vi "Command_Turret_AutoTarget.vi"(7 "Startup":bool, 8 "Timeout":dbl, 9 "Kd":dbl, 10 "Ki":dbl, 11 "Kp":dbl) -> (2 "Turret_Speed":dbl, 4 "Reint":bool, 6 "Completed":bool)   [LabVIEW 2019]
uses:
  Auto Utilities/Command_Execution_State.ctl
  Subsystems/Sensing/Sensor_Values.vi
panel:
  in  "Acceptable_Error":dbl
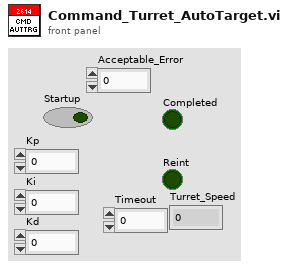
[diagram p1: front panel]
types:
  T1 = typedef "Command_Execution_State.ctl" = enum16{"Initialize", "Execute", "Finish"}
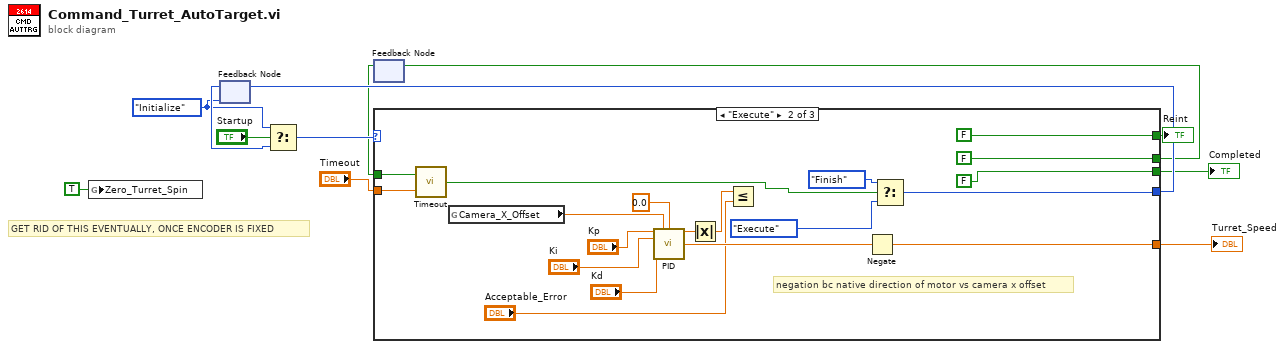
[diagram p0: block diagram]
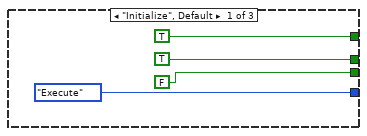
[diagram p2: hidden frame]
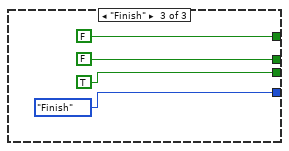
[diagram p3: hidden frame]
diagram:
  w6 = Command_Execution_State."Initialize" ("Play State")
  # "GET RID OF THIS EVENTUALLY, ONCE ENCODER IS FIXED"
  n1 = global write "Sensor_Values.vi" "Zero_Turret_Spin"(TRUE ("Zero_Turret_Spin")) -> ()
  n2 = feedback #1(w6) -> (w10:T1)
  n3 = Select(t=w6, s="Startup", f=w10) -> (s? t:f=w12:T1)
  n4 = feedback #2() -> (w4:bool)  [unwired: 1 in]
  n5 = case shown="\"Execute\"" w12 {
    tunnel: [Command_Execution_State."Execute" ("Play State") w27 Command_Execution_State."Finish" ("Play State")] -> w11
    tunnel: [FALSE FALSE TRUE] -> w9
    tunnel: [TRUE FALSE FALSE] -> w7
    tunnel: w4 -> [_ w31 _]
    tunnel: [TRUE FALSE FALSE] -> w5
    tunnel: "Timeout" -> [_ w29 _]
    tunnel: [_ w18 _] -> w2
    frame "Initialize", Default {
    }
    frame "Execute" {
      # "negation bc native direction of motor vs camera x offset"
      n6 = call "Timeout.vi"("Timeout"=w29, "Initialize"=w31) -> ("Timed Out?"=w17:bool)
      n7 = global read "Sensor_Values.vi" "Camera_X_Offset"() -> (w33:dbl)
      n8 = call "PID.vi"("Kp"="Kp", "Process Variable"=w33, "Goal"=0.0, "Ki"="Ki", "Kd"="Kd") -> ("Current Error"=w24:dbl, "Command"=w25:dbl)  [unwired: 8 in, 1 out]
      n9 = Absolute Value(x=w24) -> (abs(x)=w23:dbl)
      n10 = Less Or Equal?(x=w23, y="Acceptable_Error") -> ()  [unwired: 1 out]
      n11 = Negate(x=w25) -> (-x=w18:dbl)
      n12 = Select(t=Command_Execution_State."Finish" ("Play State"), s=w17, f=Command_Execution_State."Execute" ("Play State")) -> (s? t:f=w27:T1)
    }
    frame "Finish" {
    }
  }
  "Completed" <- w9
  "Reint" <- w7
  "Turret_Speed" <- w2
  n13 = feedback-in #1(w11) -> ()
  n14 = feedback-in #2(w5) -> ()
